vi "generator - csv.vi"() -> ()   [LabVIEW 2018]
uses:
  <vilib>/Utility/file.llb/Read Delimited Spreadsheet (string).vi
panel:
  out "error out 3":errorcluster
  out "error out 2":errorcluster
  out "error out":errorcluster
  # "ESP32 SHT85 - Config file generator"
  # "Fichiers \"configuration.cfg\" et \"sensors.cfg\" à copier à la racine de la carte SD pour chaque module"
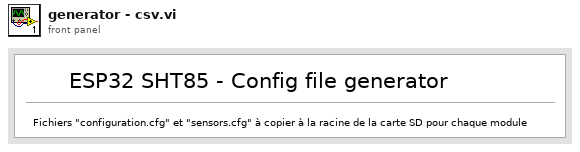
[diagram p1: front panel]
types:
  T1 = enum16{"open", "replace", "create", "open or create", "replace or create", "replace or create with confirmation"}
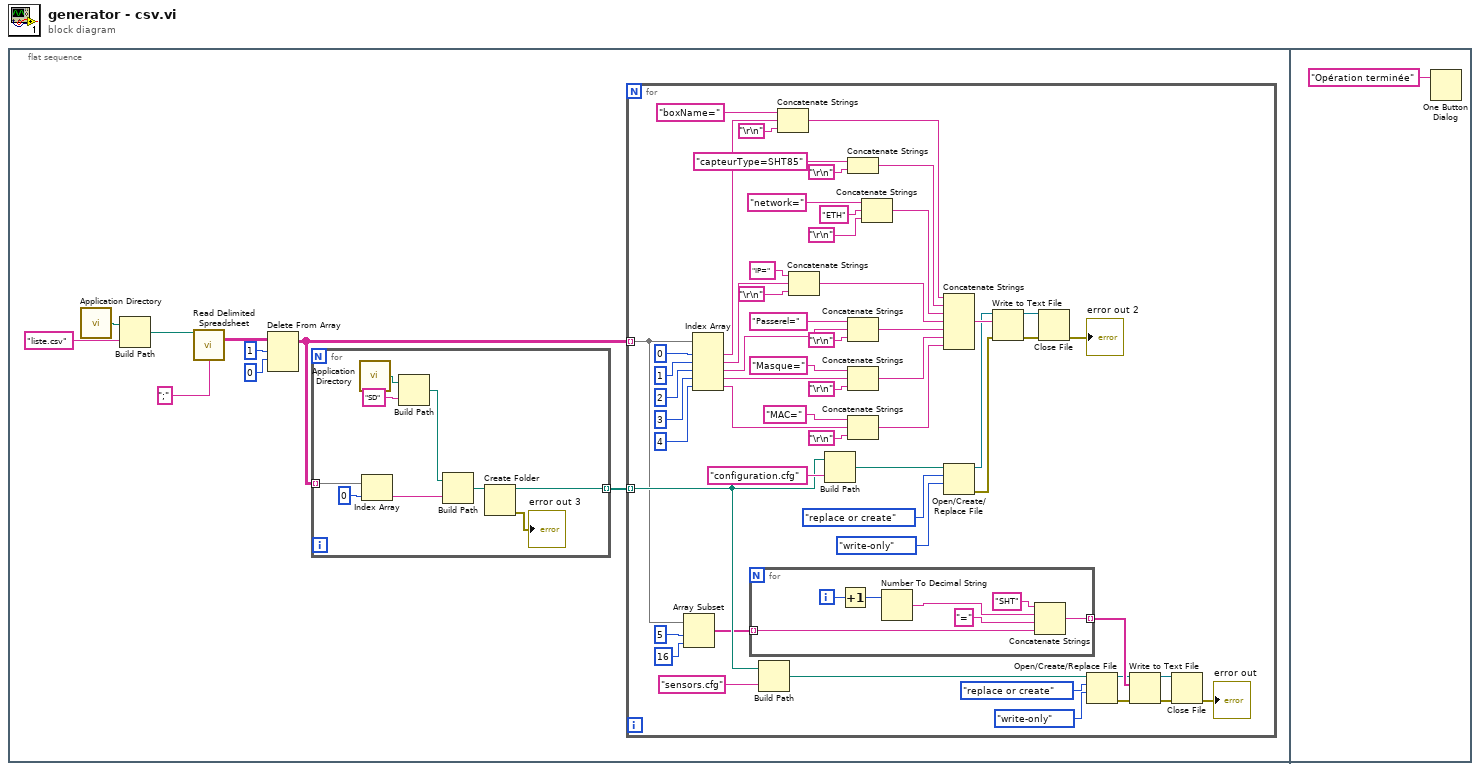
[diagram p0: block diagram]
diagram:
  n1 = flat-sequence {
    frame #0 {
      n2 = call <vilib>:"Application Directory.vi"() -> ("Application Directory"=w7:path)
      n3 = Build Path(base path=w7, name or relative path="liste.csv") -> (appended path=w8:path)
      n4 = call-poly <vilib>:"Read Delimited Spreadsheet.vi"("file path (dialog if empty)"=w8, "delimiter (\\t)"=";" ("delimiter (\\t)")) -> ("all rows"=w4:string[][])  [unwired: 8 in, 5 out]
      n5 = Delete From Array(array=w4, length=1, index (row)=0) -> (array with subset deleted=w1:string[][])  [unwired: 1 in, 1 out]
      n6 = for {
        tunnel: w1 -> [w18] mode=indexing
        tunnel: [w14] -> w5 mode=indexing
        n7 = call <vilib>:"Application Directory.vi"() -> ("Application Directory"=w13:path)
        n8 = Index Array(array=w18, index=0) -> (element=w16:string)
        n9 = Build Path(base path=w13, name or relative path="SD") -> (appended path=w11:path)
        n10 = Build Path(base path=w11, name or relative path=w16) -> (appended path=w15:path)
        n11 = Create Folder(path (use dialog)=w15) -> (created path=w14:path, error out=→"error out 3":errorcluster)  [unwired: 2 in, 1 out]
      }
      n12 = for {
        tunnel: w5 -> [w33] mode=indexing
        tunnel: w1 -> [w22] mode=indexing
        n13 = Array Subset(array=w22, index=5, length=16) -> (w19:string[])
        n14 = Index Array(array=w22, index #1=0, index #2=1, index #3=2, index #4=3, index #5=4) -> (element #1=w27:string, element #2=w26:string, element #3=w25:string, element #4=w24:string, element #5=w23:string)
        n15 = for {
          tunnel: w19 -> [w81] mode=indexing
          tunnel: [w76] -> w66 mode=indexing
          i -> [w80]
          n16 = Increment(x=w80) -> (x+1=w79:i32)
          n17 = Number To Decimal String(number=w79) -> (decimal integer string=w77:string)  [unwired: 1 in]
          n18 = Concatenate Strings("SHT", w77, "=", w81) -> (w76:string)
        }
        n19 = Build Path(base path=w33, name or relative path="sensors.cfg") -> (appended path=w75:path)
        n20 = Concatenate Strings("boxName=", w27, "\r\n") -> (w41:string)
        n21 = Concatenate Strings("IP=", w26, "\r\n") -> (w38:string)
        n22 = Build Path(base path=w33, name or relative path="configuration.cfg") -> (appended path=w74:path)
        n23 = Concatenate Strings("capteurType=SHT85", "\r\n") -> (w40:string)
        n24 = Concatenate Strings("Passerel=", w25, "\r\n") -> (w37:string)
        n25 = Concatenate Strings("Masque=", w24, "\r\n") -> (w36:string)
        n26 = Concatenate Strings("MAC=", w23, "\r\n") -> (w35:string)
        n27 = Concatenate Strings("network=", "ETH" ("string"), "\r\n") -> (w39:string)
        n28 = Concatenate Strings(w41, w40, w39, w38, w37, w36, w35) -> (w67:string)
        n29 = Open/Create/Replace File(file path (use dialog)=w74, operation (0:open)=T1."replace or create", access (0:read/write)=enum16{"read/write", "read-only", "write-only"}."write-only") -> (refnum out=w64:refnum<file>, error out=w59:errorcluster)  [unwired: 3 in, 1 out]
        n30 = Write to Text File(file (use dialog)=w64, text=w67, error in=w59) -> (refnum out=w60:refnum<file>, error out=w61:errorcluster)  [unwired: 1 in, 1 out]
        n31 = Close File(refnum=w60, error in=w61) -> (error out=→"error out 2":errorcluster)  [unwired: 1 out]
        n32 = Open/Create/Replace File(file path (use dialog)=w75, operation (0:open)=T1."replace or create", access (0:read/write)=enum16{"read/write", "read-only", "write-only"}."write-only") -> (refnum out=w65:refnum<file>, error out=w58:errorcluster)  [unwired: 3 in, 1 out]
        n33 = Write to Text File(file (use dialog)=w65, text=w66, error in=w58) -> (refnum out=w62:refnum<file>, error out=w63:errorcluster)  [unwired: 1 in, 1 out]
        n34 = Close File(refnum=w62, error in=w63) -> (error out=→"error out":errorcluster)  [unwired: 1 out]
      }
    }
    frame #1 {
      n35 = One Button Dialog(message="Opération terminée") -> ()  [unwired: 1 in, 1 out]
    }
  }
